vi "Img Unflatten RGBA Pixmap.vi"(10 "BG Color":u32(colorbox), 11 "image data":T1) -> (3 "24-bit pixmap":u32[][](array[numeric]) format="%x")   [LabVIEW 2018, in "Image Process.lvclass"]
doc: "Converts a cluster of image data into a 2D array."
uses:
  Image Process.lvclass
  <vilib>/picture/picture.llb/imagedata.ctl
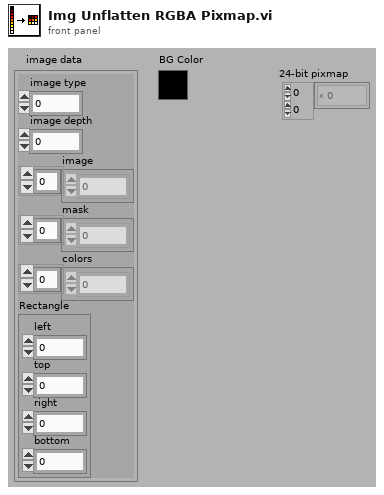
[diagram p1: front panel]
types:
  T1 = typedef "imagedata.ctl" = cluster{"image type":i32, "image depth":i32, "image":u8[], "mask":u8[], "colors":u32[], "Rectangle":cluster{"left":i16, "top":i16, "right":i16, "bottom":i16}}
  T2 = cluster{"left":i16, "top":i16, "right":i16, "bottom":i16}
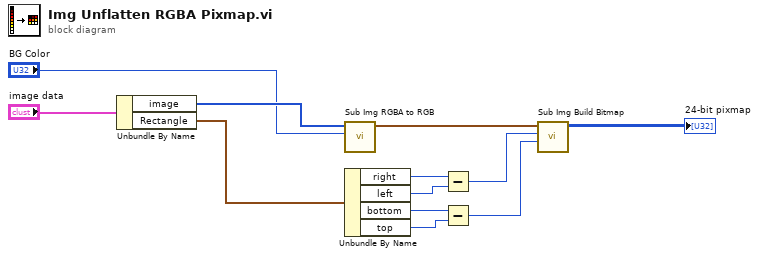
[diagram p0: block diagram]
diagram:
  n1 = Unbundle By Name("image data") -> ("image"=w2:u8[], "Rectangle"=w11:T2)
  n2 = call "Sub Img RGBA to RGB.vi"("Default Color"="BG Color", "RGBA Array"=w2) -> ("RGB Array"=w9:cluster{"R":u8, "G":u8, "B":u8}[])  [unwired: 9 in]
  n3 = Unbundle By Name(w11) -> ("right"=w8:i16, "left"=w7:i16, "bottom"=w6:i16, "top"=w5:i16)
  n4 = Subtract(x=w8, y=w7) -> (x-y=w4:i16)
  n5 = Subtract(x=w6, y=w5) -> (x-y=w3:i16)
  n6 = call "Sub Img Build Bitmap.vi"("Height"=w3, "Width"=w4, "RGB Array"=w9) -> ("24-bit pixmap"=→"24-bit pixmap":u32[][])  [unwired: 8 in]
